vi "Ejercicios Array 2.vi"() -> ()   [LabVIEW 2010]
panel:
  out "Indice 5":dbl[](array[numeric])
  out "Array + 1000":dbl[](array[numeric])
  out "Ultimas 5 casillas":dbl[](array[numeric])
  out "Array x 2":dbl[](array[numeric])
  in  "stop":bool
  out "Indice":dbl
  out "Min":dbl
  out "Indice":dbl
  out "Max":dbl
  out "Array":dbl[](array[numeric])
  in  "Array":dbl[](array[numeric])
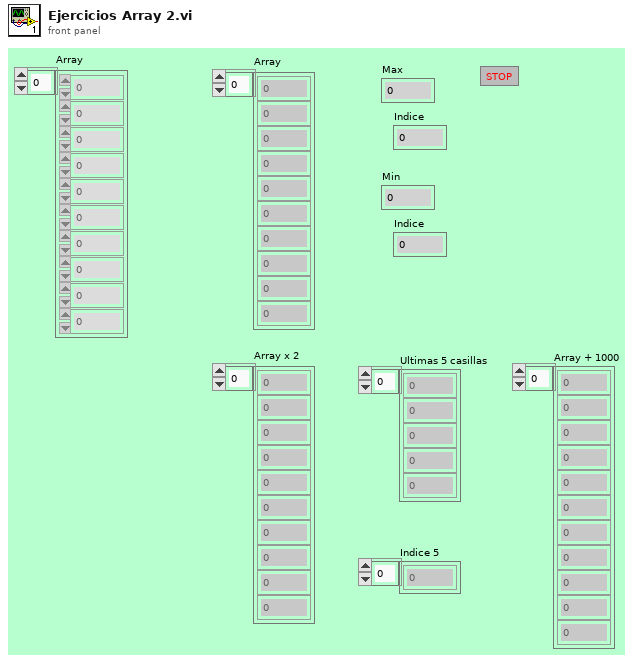
[diagram p1: front panel]
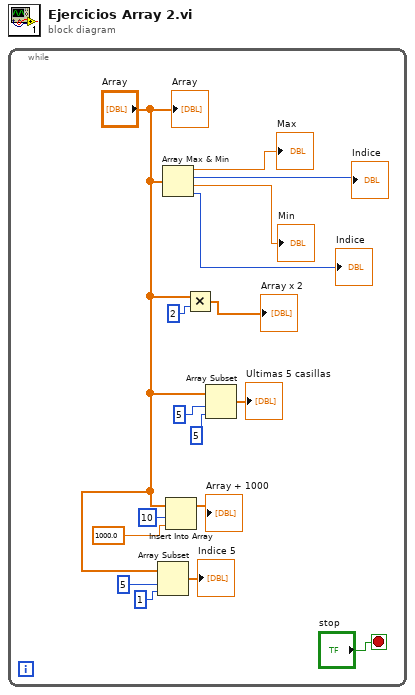
[diagram p0: block diagram]
diagram:
  n1 = while {
    stop <- "stop" stop-if-true
    n2 = Array Subset(array="Array", index=5, length=1) -> (→"Indice 5":dbl[])
    n3 = Array Max & Min(array="Array") -> (max value=→"Max":dbl, max index (indices)=→"Indice":i32, min value=→"Min":dbl, min index (indices)=→"Indice":i32)
    n4 = Insert Into Array(array="Array", index=10, new element=1000.0 ("Numeric")) -> (→"Array + 1000":dbl[])
    n5 = Multiply(x="Array", y=2) -> (x*y=→"Array x 2":dbl[])
    n6 = Array Subset(array="Array", index=5, length=5) -> (→"Ultimas 5 casillas":dbl[])
    "Array" <- "Array"
  }
